vi "CA.vi"(0 "init input ports":u8[](array[numeric]), 1 "Alg states":cluster{u32, u8}[](array[cluster]), 5 "output":u8[](array[numeric]), 7 "input ALG msg array":T1(array[cluster]), 9 "Output ALG msg array":T1(array[cluster]), 11 "VOC output msg CASHE":T1(array[cluster])) -> (3 "Output Alg states":cluster{u32, u8}[](array[cluster]), 4 "input ports":u8[](array[numeric]), 6 "modified output ports":u8[](array[numeric]), 8 "Clear input msg Array":T1(array[cluster]), 10 "ALG output array":T1(array[cluster]))   [LabVIEW 2009]
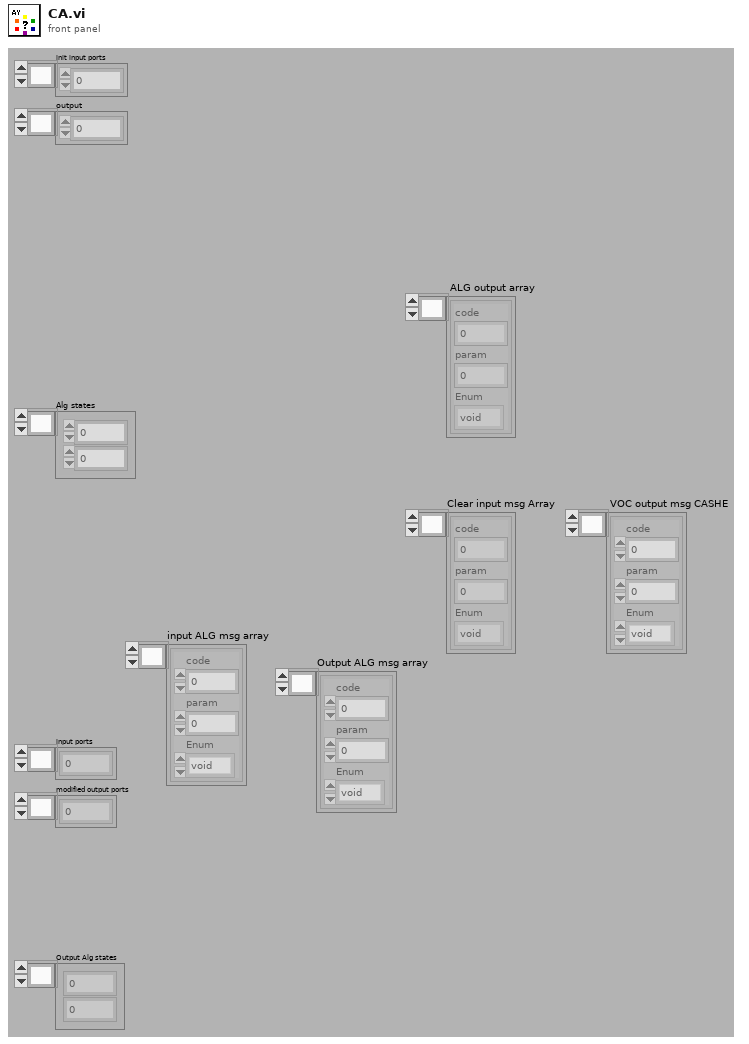
[diagram p1: front panel]
types:
  T1 = cluster{"code":i32, "param":i32, "Enum":enum16{"void", "byte", "int", "float"}}[]
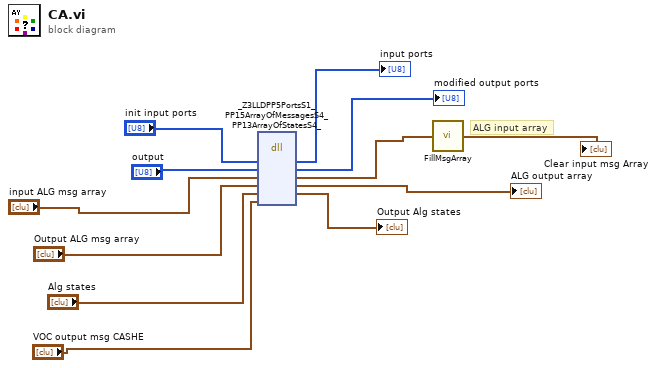
[diagram p0: block diagram]
diagram:
  # "ALG input array"
  n1 = dll-call lib="PTH1fabs CUsersUserDesktopЛях РаботаComplexOld debug progsTank PROJECTCAca.dll" fn="_Z3LLDPP5PortsS1_PP15ArrayOfMessagesS4_PP13ArrayOfStatesS4_" label="AY"("input"="init input ports", "output"="output", "msg_inp"="input ALG msg array", "msg_inp"="Output ALG msg array", "states"="Alg states", "voc_msg"="VOC output msg CASHE") -> ("input"=→"input ports":u8[], "output"=→"modified output ports":u8[], "msg_inp"=w7:T1, "msg_inp"=→"ALG output array":T1, "states"=→"Output Alg states":cluster{u32, u8}[])  [unwired: 5 in, 2 out]
  n2 = call "FillMsgArray.vi"("Input VOC msg Array"=w7) -> ("Clear msg Array"=→"Clear input msg Array":T1)
